vi "Array String(ms) to Stamp.vi"(5 "time string(ms)":string[](array[string])) -> (2 "time stamp(ms)":timestamp[](array[timestamp]))   [LabVIEW 2020]
panel:
  # "转换后有可能出现1ms差"
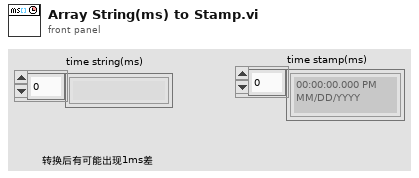
[diagram p1: front panel]
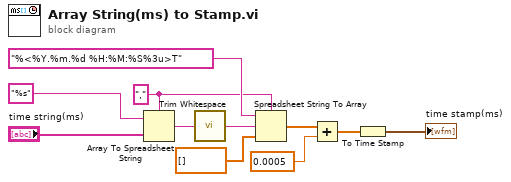
[diagram p0: block diagram]
diagram:
  w7 = "," ("delimiter (Tab)")
  n1 = Array To Spreadsheet String(delimiter (Tab)=w7, array="time string(ms)", 3:"%s" ("format string")) -> (spreadsheet string=w9:string)
  n2 = call <vilib>:"Trim Whitespace.vi"("string"=w9) -> ("trimmed string"=w8:string)  [unwired: 1 in]
  n3 = Spreadsheet String To Array(delimiter (Tab)=w7, format string="%<%Y.%m.%d %H:%M:%S%3u>T", spreadsheet string=w8, array type (2D Dbl)=dbl[] []) -> (array=w4:dbl[])
  n4 = Add(x=w4, y=0.0005 ("Numeric")) -> (x+y=w2:dbl[])
  n5 = To Time Stamp(1:w2) -> (0:→"time stamp(ms)":timestamp[])
